vi "Insert Panel into SubPanel.vi"(8 "error in (no error)":errorcluster, 9 "SubPanel":refnum<vi>, 10 "Panel In":refnum<class "Panel.lvclass">, 11 "Manager in":refnum<class "Manager.lvclass">) -> (0 "error out":errorcluster, 2 "Panel":refnum<class "Panel.lvclass">, 3 "Manager out":refnum<class "Manager.lvclass">)   [LabVIEW 2020, in "OOPanel.lvlib" / "Manager.lvclass"]
uses:
  Manager.lvclass
  Panel/Panel.lvclass
  Manager.lvclass/Manager.ctl
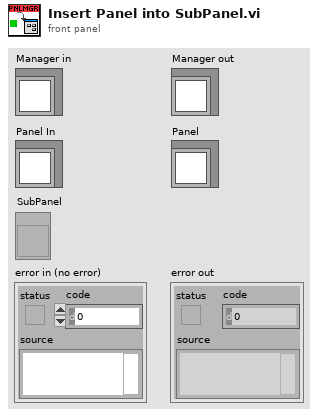
[diagram p1: front panel]
types:
  T1 = typedef "OOPanel.lvlib/Visibility State.ctl" = enum16{"Idle", "Closed", "Hidden", "Visible", "Subpanel", "Hidden Subpanel"}
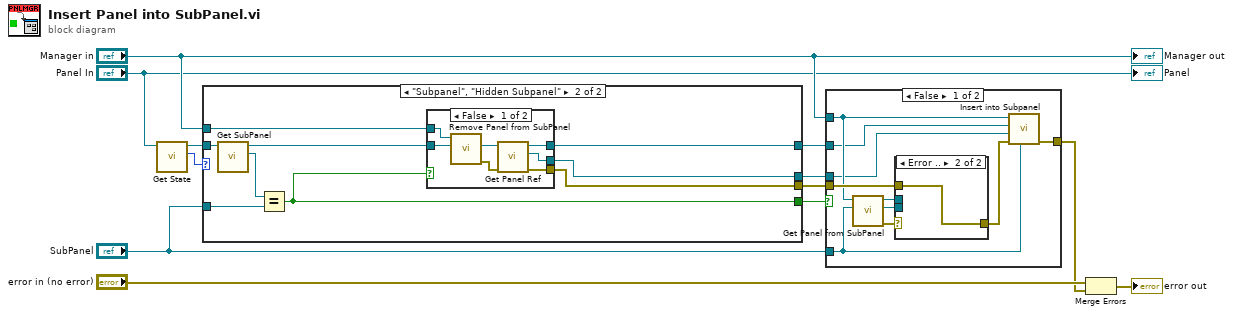
[diagram p0: block diagram]
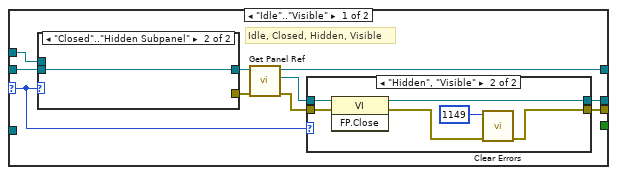
[diagram p2: hidden frame]
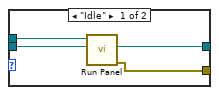
[diagram p4: hidden frame]
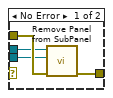
[diagram p6: hidden frame]
diagram:
  n1 = call "Get State.vi"("Panel in"="Panel In") -> ("State"=w10:T1, "Panel out"=w11:refnum<class "Panel.lvclass">)  [unwired: 8 in, 1 out]
  n2 = case shown="\"Subpanel\", \"Hidden Subpanel\"" w10 {
    selector: w10 -> [w13 _]
    tunnel: w11 -> [w22 w40]
    tunnel: "Manager in" -> [w21 w44]
    tunnel: [w16 w41] -> w3
    tunnel: [w15 w42] -> w8
    tunnel: [w14 w43] -> w9
    tunnel: "SubPanel" -> [_ w39]
    tunnel: [_ w37] -> w5
    frame "Idle".."Visible" {
      # "Idle, Closed, Hidden, Visible"
      n3 = case shown="\"Closed\"..\"Hidden Subpanel\"" w13 {
        tunnel: w22 -> [w34 w35]
        tunnel: w21 -> [w33 _]
        tunnel: [w32 w35] -> w20
        tunnel: [w31 _] -> w19
        frame "Idle" {
          n4 = call "Run Panel.vi"("Panel In"=w34, "Manager in"=w33) -> ("error out"=w31:errorcluster, "Panel"=w32:refnum<class "Panel.lvclass">)  [unwired: 7 in, 1 out]
        }
        frame "Closed".."Hidden Subpanel" {
        }
      }
      n5 = call "Get Panel Ref.vi"("error in (no error)"=w19, "Panel in"=w20) -> ("error out"=w18:errorcluster, "Panel Ref"=w17:refnum<vi>, "Panel out"=w14:refnum<class "Panel.lvclass">)  [unwired: 7 in]
      n6 = case shown="\"Hidden\", \"Visible\"" w13 {
        tunnel: w18 -> [w23 w30]
        tunnel: w17 -> [w24 w29]
        tunnel: [w23 w27] -> w16
        tunnel: [w24 w28] -> w15
        frame "Idle", "Closed", "Subpanel", "Hidden Subpanel" {
        }
        frame "Hidden", "Visible" {
          n7 = invoke class="VI" method="FP.Close"(reference=w29, error in=w30) -> (reference out=w28:refnum<vi>, error out=w25:errorcluster)  [unwired: 1 in, 1 out]
          n8 = call <vilib>:"Clear Errors.vi"("error in (no error)"=w25, "specific error code to clear (0: all)"=1149) -> ("error out"=w27:errorcluster)  [unwired: 4 in, 1 out]
        }
      }
    }
    frame "Subpanel", "Hidden Subpanel" {
      n9 = call "Get SubPanel.vi"("Panel in"=w40) -> ("SubPanel"=w38:refnum<vi>, "Panel out"=w36:refnum<class "Panel.lvclass">)  [unwired: 8 in, 1 out]
      n10 = Equal?(x=w38, y=w39) -> (x = y?=w37:bool)
      n11 = case shown="False" w37 {
        tunnel: w44 -> [w51 _]
        tunnel: [w49 _] -> w43
        tunnel: [w48 _] -> w42
        tunnel: [w46 _] -> w41
        tunnel: w36 -> [w45 _]
        frame False {
          n12 = call "Remove Panel from SubPanel.vi"("Panel In"=w45, "Manager in"=w51) -> ("error out"=w47:errorcluster, "Panel"=w50:refnum<class "Panel.lvclass">)  [unwired: 7 in, 1 out]
          n13 = call "Get Panel Ref.vi"("error in (no error)"=w47, "Panel in"=w50) -> ("error out"=w46:errorcluster, "Panel Ref"=w48:refnum<vi>, "Panel out"=w49:refnum<class "Panel.lvclass">)  [unwired: 7 in]
        }
        frame True {
        }
      }
    }
  }
  n14 = case shown="False" w5 {
    tunnel: "Manager in" -> [w57 _]
    tunnel: w9 -> [w56 _]
    tunnel: "SubPanel" -> [w55 _]
    tunnel: w8 -> [w54 _]
    tunnel: w3 -> [w58 w67]
    tunnel: [w52 w67] -> w1
    frame False {
      n15 = call "Get Panel from SubPanel.vi"("SubPanel"=w55, "Manager in"=w57) -> ("error out"=w60:errorcluster, "Panel"=w61:refnum<class "Panel.lvclass">, "Manager out"=w59:refnum<class "Manager.lvclass">)  [unwired: 6 in, 1 out]
      n16 = case shown="Error .." w60 {
        tunnel: w61 -> [w63 _]
        tunnel: w59 -> [w64 _]
        tunnel: [w62 w66] -> w53
        tunnel: w58 -> [w65 w66]
        frame No Error {
          n17 = call "Remove Panel from SubPanel.vi"("error in (no error)"=w65, "Panel In"=w63, "Manager in"=w64) -> ("error out"=w62:errorcluster)  [unwired: 6 in, 2 out]
        }
        frame Error {
        }
      }
      n18 = call "Insert into Subpanel.vi"("SubPanel"=w55, "error in (no error)"=w53, "VI"=w54, "Panel"=w56, "Manager in"=w57) -> ("error out"=w52:errorcluster)  [unwired: 5 in, 1 out]
    }
    frame True {
      # "Panel already in subpanel."
    }
  }
  n19 = Merge Errors("error in (no error)", w1) -> (→"error out":errorcluster)
  "Manager out" <- "Manager in"
  "Panel" <- "Panel In"
